vi "SectionA.vi"() -> ()   [LabVIEW 2010]
uses:
  <vilib>/Utility/file.llb/Write To Spreadsheet File (DBL).vi
  <vilib>/Analysis/NI_AALBase.lvlib
panel:
  in  "Path":path
  in  "Iterations":dbl format="%.2f"
  out "XY Graph 2":cluster{dbl[], dbl[]}(graph)
  out "XY Graph":cluster{dbl[], dbl[]}(graph)
  out "Numeric 2":dbl format="%.2f"
  out "error out 2":errorcluster
  out "data":string
  out "Numeric":dbl format="%.2f"
  in  "Step":dbl format="%.2f"
  in  "error in (no error)":errorcluster
  in  "Wait/s":dbl format="%.2f"
  in  "Stop 3":dbl format="%.2f"
  in  "Stop 2":dbl format="%.2f"
  in  "Stop 1":dbl format="%.2f"
  in  "Start 3":dbl format="%.2f"
  in  "Start 2":dbl format="%.2f"
  in  "Start 1":dbl format="%.2f"
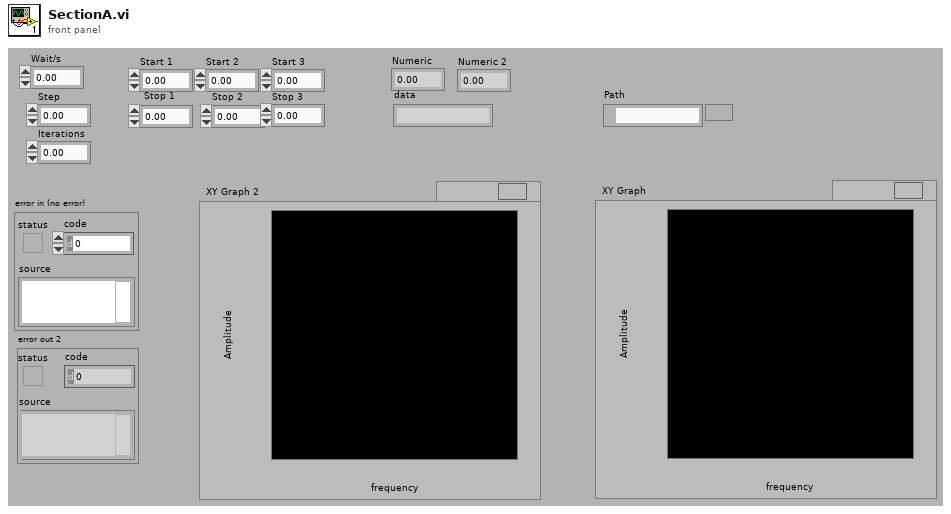
[diagram p1: front panel]
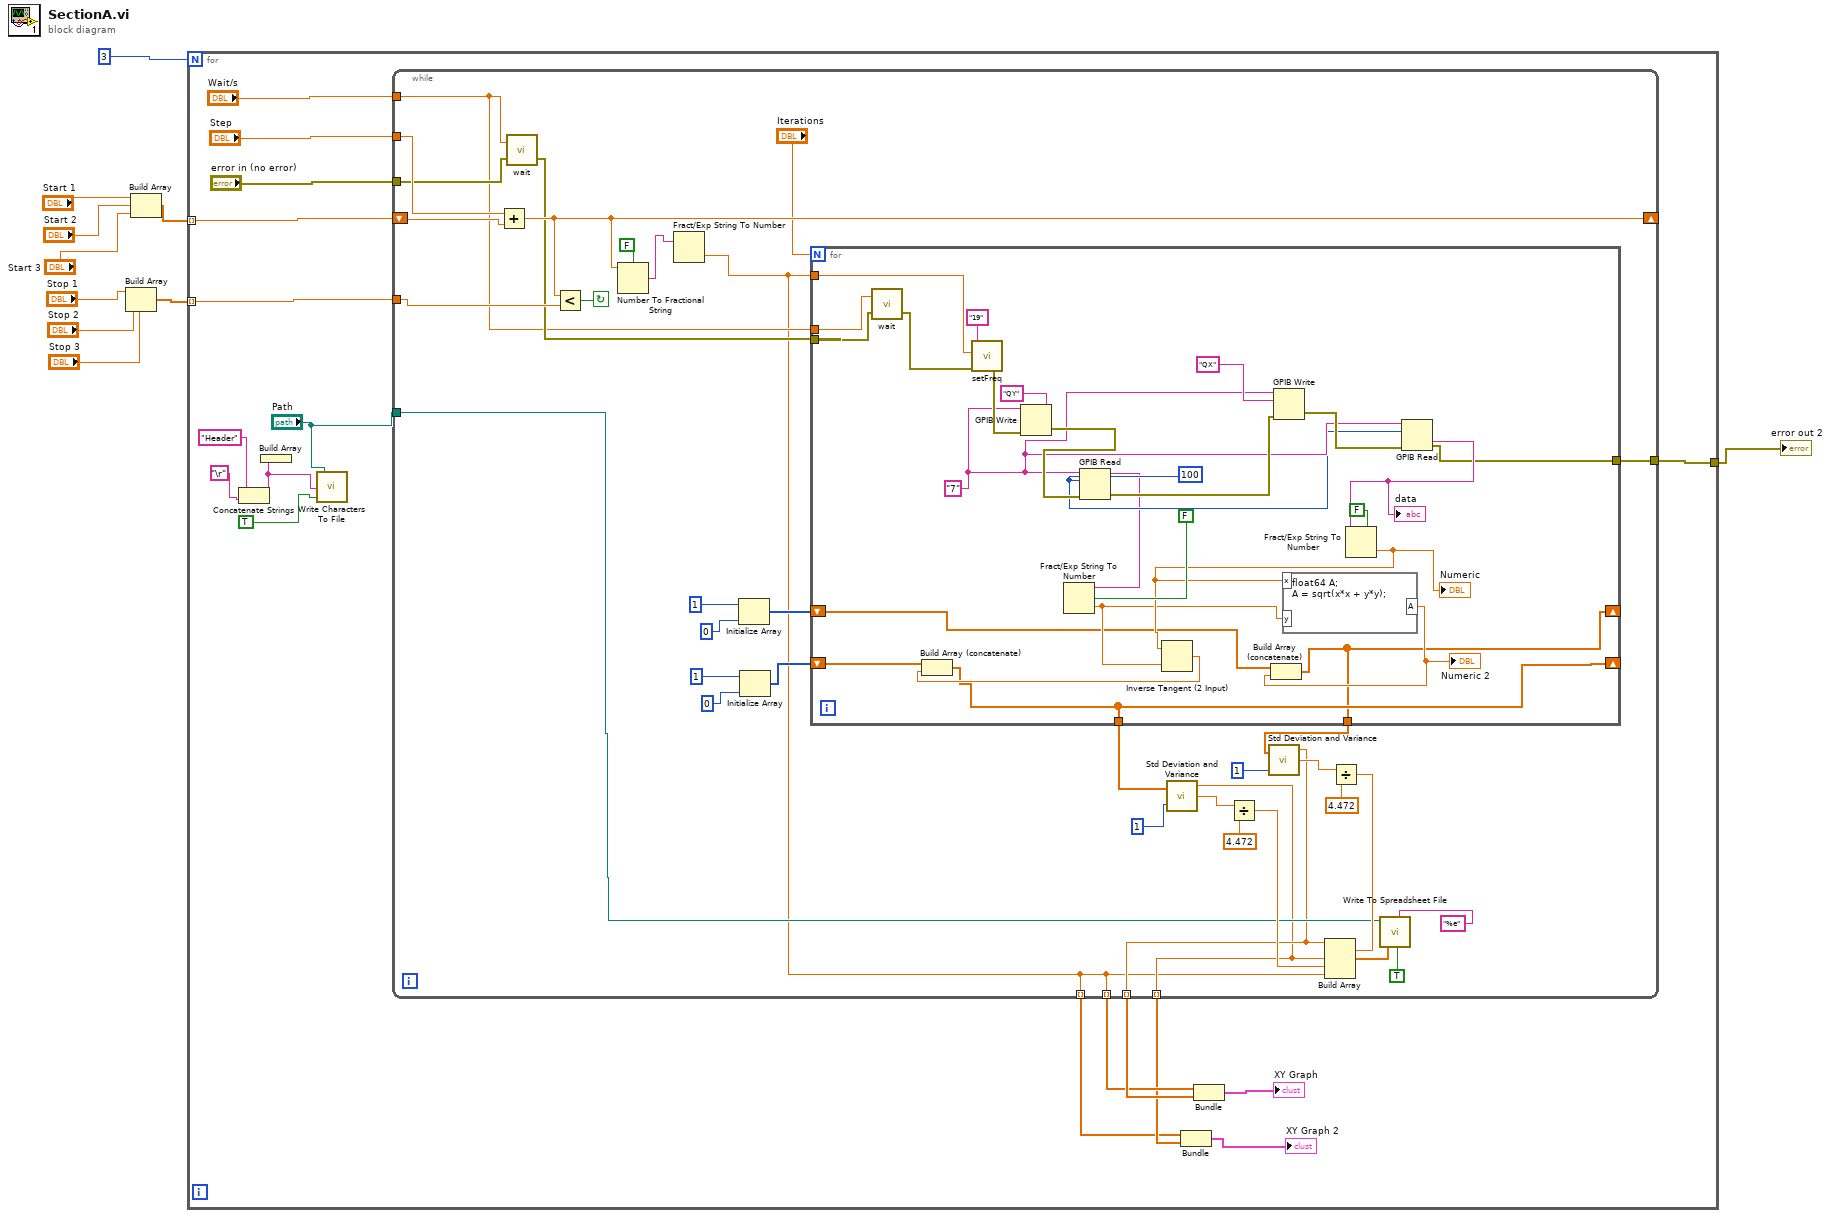
[diagram p0: block diagram]
diagram:
  n1 = Build Array("Stop 1", "Stop 2", "Stop 3") -> (w3:dbl[])
  n2 = Build Array("Start 1", "Start 2", "Start 3") -> (w4:dbl[])
  n3 = for {
    N: 3 -> [_]
    tunnel: w4 -> [w27] mode=indexing
    tunnel: w3 -> [w26] mode=indexing
    tunnel: [w22] -> w1
    n4 = Concatenate Strings("Header", "\r") -> (w16:string)
    n5 = Build Array(w16) -> ()  [unwired: 1 out]
    n6 = call <vilib>:"Write Characters To File.vi"("append to file? (new file:F)"=TRUE, "character string"=w16, "file path (dialog if empty)"="Path") -> ()  [unwired: 2 in, 1 out]
    n7 = while {
      tunnel: "Path" -> [w34]
      tunnel: w26 -> [w57]
      tunnel: "Step" -> [w61]
      tunnel: "Wait/s" -> [w53]
      tunnel: "error in (no error)" -> [w60]
      shift-right: [w55] -> _
      shift-left: w27 -> [w62]
      tunnel: [w52] -> w22
      tunnel: [w31] -> w14 mode=indexing
      tunnel: [w29] -> w13 mode=indexing
      tunnel: [w30] -> w12 mode=indexing
      tunnel: [w29] -> w11 mode=indexing
      stop <- w56 continue-if-true
      n8 = Add(x=w61, y=w62) -> (x+y=w55:dbl)
      n9 = call "wait.vi"("error in"=w60, "Wartezeit in Sek"=w53) -> ("error out"=w54:errorcluster)  [unwired: 1 in]
      n10 = Less?(x=w55, y=w57) -> (x < y?=w56:bool)
      n11 = Number To Fractional String(use system decimal point (T)=FALSE, number=w55) -> (F-format string=w59:string)  [unwired: 2 in]
      n12 = Fract/Exp String To Number(string=w59) -> (number=w29:dbl)  [unwired: 3 in, 1 out]
      n13 = Initialize Array(1, 0) -> (w35:i32[])
      n14 = Initialize Array(1, 0) -> (w36:i32[])
      n15 = for {
        N: "Iterations" -> [_]
        tunnel: w54 -> [w87]
        tunnel: w53 -> [w88]
        tunnel: w29 -> [w72]
        tunnel: [w71] -> w52
        shift-right: [w63] -> _
        shift-left: w35 -> [w65]
        shift-right: [w64] -> _
        shift-left: w36 -> [w66]
        tunnel: [w64] -> w33
        tunnel: [w63] -> w32
        w78 = 100
        w79 = "7"
        n16 = call "wait.vi"("error in"=w87, "Wartezeit in Sek"=w88) -> ("error out"=w73:errorcluster)  [unwired: 1 in]
        n17 = call "setFreq.vi"("error in"=w73, "Frequenz in Hz"=w72, "address string"="19") -> ("error out"=w83:errorcluster)  [unwired: 3 in]
        n18 = GPIB Write(0:w79, 1:"QY", 3:w83) -> (6:w84:errorcluster)  [unwired: 2 in, 1 out]
        n19 = GPIB Read(0:w79, 1:w78, 3:w84) -> (5:w77:string, 7:w81:errorcluster)  [unwired: 2 in, 1 out]
        n20 = Fract/Exp String To Number(use system decimal point (T)=FALSE, string=w77) -> (number=w69:dbl)  [unwired: 2 in, 1 out]
        n21 = GPIB Write(0:w79, 1:"QX", 3:w81) -> (6:w80:errorcluster)  [unwired: 2 in, 1 out]
        n22 = GPIB Read(0:w79, 1:w78, 3:w80) -> (5:w76:string, 7:w71:errorcluster)  [unwired: 2 in, 1 out]
        "data" <- w76
        n23 = Fract/Exp String To Number(use system decimal point (T)=FALSE, string=w76) -> (number=w70:dbl)  [unwired: 2 in, 1 out]
        "Numeric" <- w70
        n24 = Inverse Tangent (2 Input)(1:w69, 2:w70) -> (0:w67:dbl)
        n25 = Build Array (concatenate)(w66, w67) -> (w64:dbl[])
        n26 = formula code="float64 A;\nA = sqrt(x*x + y*y);"("x"=w70, "y"=w69) -> ("A"=w68:dbl)
        "Numeric 2" <- w68
        n27 = Build Array (concatenate)(w65, w68) -> (w63:dbl[])
      }
      n28 = call <vilib>:"Std Deviation and Variance.vi"("X"=w33, "Weighting (Sample)"=1) -> ("mean"=w30:dbl, "standard deviation"=w46:dbl)  [unwired: 1 out]
      n29 = Divide(x=w46, y=4.472) -> (x/y=w44:dbl)
      n30 = call <vilib>:"Std Deviation and Variance.vi"("X"=w32, "Weighting (Sample)"=1) -> ("mean"=w31:dbl, "standard deviation"=w49:dbl)  [unwired: 1 out]
      n31 = Divide(x=w49, y=4.472) -> (x/y=w47:dbl)
      n32 = Build Array(w31, w47, w30, w44, w29) -> (w43:dbl[])
      n33 = call-poly <vilib>:"Write To Spreadsheet File.vi"("format (%.3f)"="%e", "append to file? (new file:F)"=TRUE, "1D data"=w43, "file path (dialog if empty)"=w34) -> ()  [unwired: 4 in, 1 out]
    }
    n34 = Bundle(w11, w12) -> (→"XY Graph 2":cluster{dbl[], dbl[]})  [unwired: 1 in]
    n35 = Bundle(w13, w14) -> (→"XY Graph":cluster{dbl[], dbl[]})  [unwired: 1 in]
  }
  "error out 2" <- w1
